vi "WPI_SimpleGyro_Open.vi"(8 "error in":errorcluster, 10 "Sample Rate (ms)":dbl=0.5, 11 "SPI Chip Select":T3=enum."SPI On-Board, CS2") -> (0 "error out":errorcluster, 3 "SimpleGyroDevRef":T1)   [LabVIEW 2014, in "SimpleGyro.lvlib"]
doc: "Initiates communication between a SimpleGyro and the RoboRIO."
uses:
  SimpleGyro.lvlib
  <vilib>/Rock Robotics/SystemInterfaces/spilib/spi_bus.ctl
  WPI_SimpleGyroDevRef.ctl
  <vilib>/Rock Robotics/SystemInterfaces/Typedef/FPGA_TypedefDigitalModule.ctl
  <vilib>/Rock Robotics/WPI/SPI/WPI_SPIMode.ctl
  WPIlib ADXRS453/WPI_Gyro_ADXRS453_Registers.ctl
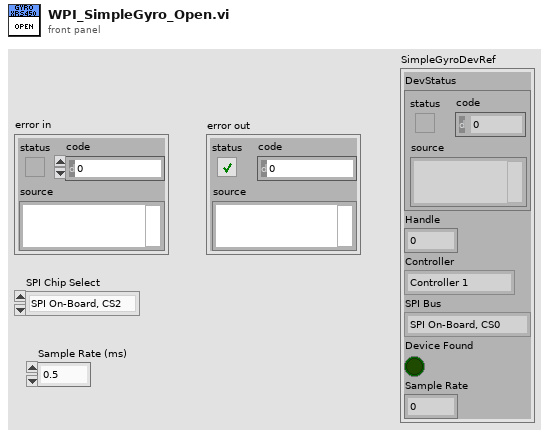
[diagram p1: front panel]
types:
  T1 = typedef "SimpleGyro.lvlib/WPI_SimpleGyroDevRef.ctl" = cluster{"DevStatus":errorcluster, "Handle":i32, "Controller":T2, "SPI Bus":T3, "Device Found":bool, "Sample Rate":dbl}
  T2 = typedef "FPGA_TypedefDigitalModule.ctl" = enum16{"Controller 1"}
  T3 = typedef "spi_bus.ctl" = enum16{"SPI On-Board, CS0", "SPI On-Board, CS1", "SPI On-Board, CS2", "SPI On-Board, CS3", "SPI MXP", "Invalid"}
  T4 = typedef "WPI_SPIMode.ctl" = enum16{"Mode 0 (Clk Idle Low,Sample on Leading)", "Mode 1 (Clk Idle Low,Sample on Trailing)", "Mode 2 (Clk Idle High,Sample on Leading)", "Mode 3 (Clk Idle High,Sample on Trailing)"}
  T5 = typedef "SimpleGyro.lvlib/WPI_Gyro_ADXRS453_Registers.ctl" = u16
  T6 = typedef "WPI_SPIDevRef.ctl" = cluster{"DevStatus":errorcluster, "Handle":i32, "Controller":T2, "SPI Bus":T3}
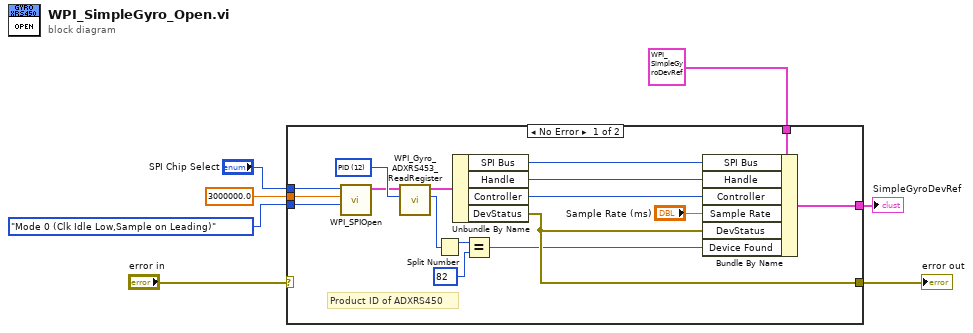
[diagram p0: block diagram]
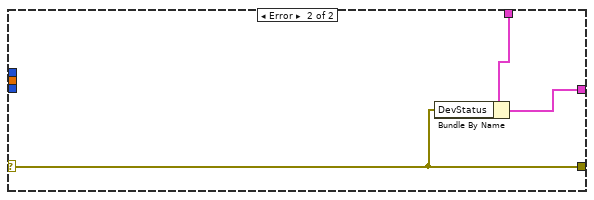
[diagram p2: hidden frame]
diagram:
  n1 = case shown="No Error" "error in" {
    selector: "error in" -> [_ w26]
    tunnel: "SPI Chip Select" -> [w24 _]
    tunnel: 3000000.0 ("Clock Rate (Hz)") -> [w23 _]
    tunnel: WPI_SPIMode."Mode 0 (Clk Idle Low,Sample on Leading)" ("Mode (3)") -> [w22 _]
    tunnel: [w16 w26] -> w3
    tunnel: T1 {"DevStatus"={"status"=FALSE, "code"=0, "source"=""}, "Handle"=0, "Controller"=enum."Controller 1", "SPI Bus"=enum."SPI On-Board, CS0", "Device Found"=FALSE, "Sample Rate"=0.0} ("SimpleGyroDevRef 2") -> [w21 w27]
    tunnel: [w17 w25] -> w1
    frame No Error {
      w14 = T5 12 items=["Rate"=0, "Tem"=2, "LoCST"=4, "HiCST"=6, "Quad"=8, "Fault"=10, "PID"=12, "SN High"=14, "SN Low"=16]
      # "Product ID of ADXRS450"
      n2 = call <vilib>:"WPI_SPIOpen.vi"("Mode (3)"=w22, "Clock Rate (Hz)"=w23, "SPI Bus"=w24) -> ("SPIDevRef"=w10:T6)  [unwired: 7 in, 1 out]
      n3 = call "WPI_Gyro_ADXRS453_ReadRegister.vi"("ADXRS453 Register"=w14, "SPIDevRef in"=w10) -> ("Register Value"=w13:u16, "SPIDevRef out"=w9:T6)  [unwired: 7 in, 1 out]
      n4 = Split Number(x=w13) -> (hi(x)=w12:u8)  [unwired: 1 out]
      n5 = Unbundle By Name(w9) -> ("SPI Bus"=w20:T3, "Handle"=w19:i32, "Controller"=w18:T2, "DevStatus"=w16:errorcluster)
      n6 = Equal?(x=w12, y=u8 82) -> (x = y?=w8:bool)
      n7 = Bundle By Name(cluster=w21, "SPI Bus"=w20, "Handle"=w19, "Controller"=w18, "Sample Rate"="Sample Rate (ms)", "DevStatus"=w16, "Device Found"=w8) -> (w17:T1)
    }
    frame Error {
      n8 = Bundle By Name(cluster=w27, "DevStatus"=w26) -> (w25:T1)
    }
  }
  "error out" <- w3
  "SimpleGyroDevRef" <- w1
